vi "sav_dat2dbo_w.vi"(4 "ObjIds":i32[](array[numeric]), 5 "Slide Ref":refnum<vi>, 6 "Mult":i32=100000, 7 "date/time":timestamp, 8 "error in":errorcluster, 10 "Array":cluster{"x0":dbl, "dx":dbl, "y":sgl[][]}[](array[cluster]), 11 "conn ref":T1) -> (0 "error out":errorcluster, 3 "conn ref out":T1)   [LabVIEW 2010]
uses:
  <vilib>/Addons/database/Connection.llb/Conn ObjectReference.ctl
  <vilib>/addons/database/Command.llb/Cmd Execute.vi
  <vilib>/addons/database/Recordset.llb/Rec Destroy - Command.vi
  <vilib>/addons/database/Command.llb/Cmd Delete.vi
  <vilib>/addons/database/NI_Database_API.lvlib
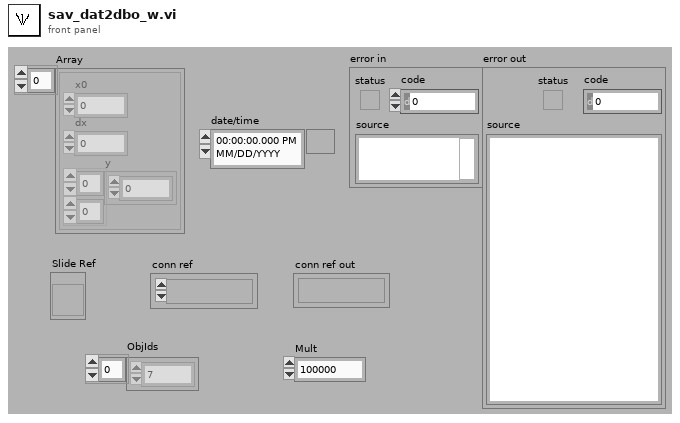
[diagram p1: front panel]
types:
  T1 = typedef "NI_Database_API.lvlib/Conn ObjectReference.ctl" = refnum<k1>
  T2 = typedef "NI_Database_API.lvlib/DB Tools Parameter Info.ctl" = cluster{"parameter name":string, "type":T3, "direction":T4, "value":variant}
  T3 = typedef "NI_Database_API.lvlib/DB Tools DataTypes.ctl" = enum16{"String", "Long (I32)", "Single (SGL)", "Double (DBL)", "Date/Time", "Binary"}
  T4 = typedef "NI_Database_API.lvlib/DB Tools Parameter Dir.ctl" = enum32{"Input", "Output", "Input/Output", "Return Value"}
  T5 = typedef "NI_Database_API.lvlib/Cmd ObjectReference.ctl" = refnum<k1>
  T6 = typedef "NI_Database_API.lvlib/Cmd-Rec Object Reference.ctl" = refnum<k1>
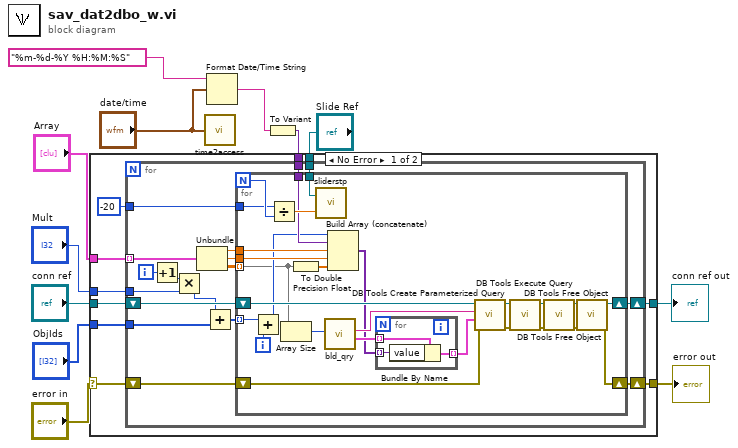
[diagram p0: block diagram]
diagram:
  n1 = call "time2access.vi"("time stamp"="date/time") -> ()  [unwired: 1 out]
  n2 = Format Date/Time String(time format string (%c)="%m-%d-%Y %H:%M:%S", seconds (now)="date/time") -> (date/time string=w1:string)  [unwired: 1 in]
  n3 = To Variant(anything=w1) -> (Variant=w9:variant)
  n4 = case shown="No Error" "error in" {
    selector: "error in" -> [w13 w71]
    tunnel: "Mult" -> [w22 _]
    tunnel: "Slide Ref" -> [w21 _]
    tunnel: "conn ref" -> [w20 w70]
    tunnel: w9 -> [w18 _]
    tunnel: "Array" -> [w17 _]
    tunnel: [w16 w70] -> w7
    tunnel: [w15 w71] -> w6
    tunnel: "ObjIds" -> [w14 _]
    frame No Error {
      n5 = for {
        tunnel: w22 -> [w39]
        tunnel: w21 -> [w37]
        tunnel: -20 ("Value") -> [w28]
        tunnel: w17 -> [w27] mode=indexing
        tunnel: w14 -> [w25]
        tunnel: w18 -> [w24]
        shift-right: [w38] -> w15
        shift-left: w13 -> [w36]
        shift-right: [w34] -> w16
        shift-left: w20 -> [w35]
        i -> [w23]
        n6 = Increment(x=w23) -> (x+1=w29:i32)
        n7 = Multiply(x=w29, y=w39) -> (x*y=w26:i32)
        n8 = Unbundle(w27) -> ("x0"=w32:dbl, "dx"=w31:dbl, "y"=w33:sgl[][])
        n9 = Add(x=w26, y=w25) -> (x+y=w30:i32[])
        n10 = for {
          N -> [w64]
          tunnel: w33 -> [w41] mode=indexing
          shift-right: [w49] -> w38
          shift-left: w36 -> [w57]
          tunnel: w32 -> [w60]
          tunnel: w31 -> [w59]
          tunnel: w30 -> [w65] mode=indexing
          tunnel: w37 -> [w62]
          tunnel: w28 -> [w63]
          shift-right: [w50] -> w34
          shift-left: w35 -> [w58]
          tunnel: w24 -> [w48]
          i -> [w66]
          n11 = Add(x=w65, y=w66) -> (x+y=w42:i32)
          n12 = Divide(x=w63, y=w64) -> (x/y=w61:dbl)
          n13 = Array Size(array=w41) -> (size(s)=w47:i32)
          n14 = To Double Precision Float(number=w41) -> (double precision float=w40:dbl[])
          n15 = call "sliderstp.vi"("y"=w61, "Slide Ref"=w62) -> ()
          n16 = call "bld_qry.vi"("N"=w47) -> ("Parameters"=w45:T2[], "Query"=w46:string)  [unwired: 5 in]
          n17 = Build Array (concatenate)(w42, w48, w60, w59, w40) -> (w44:variant[])
          n18 = for {
            tunnel: w45 -> [w69] mode=indexing
            tunnel: w44 -> [w68] mode=indexing
            tunnel: [w67] -> w43 mode=indexing
            n19 = Bundle By Name(cluster=w69, "value"=w68) -> (w67:T2)
          }
          n20 = call <vilib>:"DB Tools Create Parameterized Query.vi"("error in (no error)"=w57, "parameters"=w43, "SQL query"=w46, "connection reference"=w58) -> ("error out"=w55:errorcluster, "command reference"=w56:T5)  [unwired: 3 in, 1 out]
          n21 = call-poly <vilib>:"DB Tools Execute Query.vi"("error in (no error)"=w55, "command reference"=w56) -> ("error out"=w54:errorcluster, "command-recordset reference"=w53:T6)  [unwired: 6 in]
          n22 = call-poly <vilib>:"DB Tools Free Object.vi"("error in (no error)"=w54, "command-recordset reference"=w53) -> ("error out"=w52:errorcluster, "command reference"=w51:T5)  [unwired: 8 in]
          n23 = call-poly <vilib>:"DB Tools Free Object.vi"("error in (no error)"=w52, "command reference"=w51) -> ("error out"=w49:errorcluster, "connection reference"=w50:T1)  [unwired: 8 in]
        }
      }
    }
    frame Error {
    }
  }
  "error out" <- w6
  "conn ref out" <- w7
